vi "PXF4_set_manual_MV.vi"(8 "error in":errorcluster, 10 "MV_manual":u8, 11 "Modbus Master in":refnum<class "Modbus Master.lvclass">) -> (0 "error out":errorcluster, 3 "Modbus Master out":refnum<class "Modbus Master.lvclass">)   [LabVIEW 2019]
uses:
  <vilib>/NI/Modbus Library/API/Master/Modbus Master.lvclass
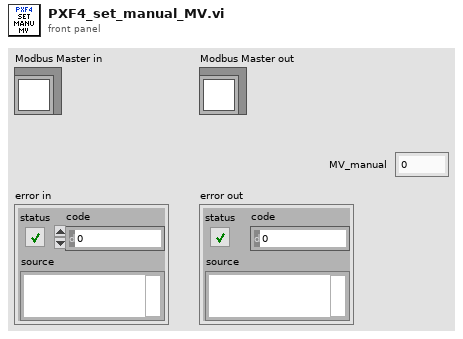
[diagram p1: front panel]
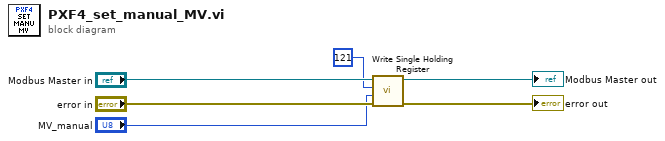
[diagram p0: block diagram]
diagram:
  n1 = call-dynamic "Write Single Holding Register.vi"("error in"="error in", "register to write"="MV_manual", "address"=u16 121, "Modbus master in"="Modbus Master in") -> ("error out"=→"error out":errorcluster, "Modbus master out"=→"Modbus Master out":refnum<class "Modbus Master.lvclass">)  [unwired: 6 in]
